vi "DCS_Dual_Inst.vi"(3 "error in":errorcluster) -> (10 "error out":errorcluster)   [LabVIEW 2013]
uses:
  <vilib>/Utility/miscctls.llb/LVPointTypeDef.ctl
  Controls/Role ID.ctl
panel:
  out "Changed front panel":bool
  in  "stop":bool
  in  "Tab Control":enum32{"Engineering Graphs", "Maintenance"}(tab)
  out "DCS 2 Second Plane":ext[][](graph)
  out "DCS 2 First Plane":ext[][](graph)
  out "DCS 1 Second Plane":ext[][](graph)
  out "DCS 1 First Plane":ext[][](graph)
  out "DCS 1 Signals":dbl[][](graph)
  out "DCS 2 Signals":dbl[][](graph)
  in  "Save Waveforms":bool
  in  "Minimum Particle Velocity (km/s)":dbl=3.0
  in  "Use Partical Veloctiy":bool=TRUE
  out "Aquisition Rate Value 2":i64
  out "Aquisition Rate Value 1":i64
  out "DAQ 1 Sample Size Window":u32
  in  "DAQ 1 Trim Time":dbl=0.0001
  in  "DAQ 2 Trim Time":dbl=0.0001
  out "DAQ 2 Sample Size Window":i32
  in  "Posttrigger size 2":i32=5000
  in  "Acquisition Rate 2":u16(ring) items=["40 MHz", "20 MHz", "10 MHz", "5 MHz", "2.5 MHz", "1 MHz", "100 kHz", "10 kHz"]
  in  "Pretrigger size 2":i32=1
  in  "Rising or falling? 2":bool
  in  "Jorger 2 TR slot":i32=6
  out "Sampling Frequency":u16(ring) items=["40 MHz", "20 MHz", "10 MHz", "5 MHz", "2.5 MHz", "1 MHz", "100 kHz", "10 kHz"]
  out "Length of Sample":dbl caption="s" format="%^#_3g"
  out "Memory Address Pointer":ext
  out "Post trigger Size":ext
  out "Pretrigger Size":ext
  out "Trigger Generation register":i32=23 format="%.0b"
  out "status register":i8=4 format="%08b"
  out "control register":i16=23 format="%015b"
  in  "Posttrigger size":i32=1
  in  "Acquisition Rate":u16(ring) items=["40 MHz", "20 MHz", "10 MHz", "5 MHz", "2.5 MHz", "1 MHz", "100 kHz", "10 kHz"]
  in  "Pretrigger size":i32=15000
  in  "Rising or falling?":bool
  out "Running Errors":errorcluster
  in  "Jorger 1 TR slot":i32=3
  in  "Joerger 1 Channels":i32[](array[numeric])=[0, 1, 2, 3, 4, 5, 6, 9]
  in  "Joerger 2 Channels":i32[](array[numeric])=[0, 1, 2, 3, 4, 6, 7, 8]
  out "control register 2":i16=23 format="%015b"
  out "status register 2":i8=4 format="%08b"
  out "Memory Address Pointer 2":ext
  out "Post trigger Size 2":ext
  out "Pretrigger Size 2":ext
  out "Sampling Frequency 2":u16(ring) items=["40 MHz", "20 MHz", "10 MHz", "5 MHz", "2.5 MHz", "1 MHz", "100 kHz", "10 kHz"]
  out "DCS_1_Pre_Trigger":dbl
  out "DCS_2_Post_Trigger":dbl
  # "Ensure Joeger Card Channels are functional.\nDefault values should reflect this."
  # "Rising or falling? not functional. Ignore"
  # "DAQ 2 Parameter Controls"
  # "Falling"
  # "Rising"
  # "DAQ Parameter Indicators"
  # "DAQ 1 Parameter Controls"
  # "Falling"
  # "Rising"
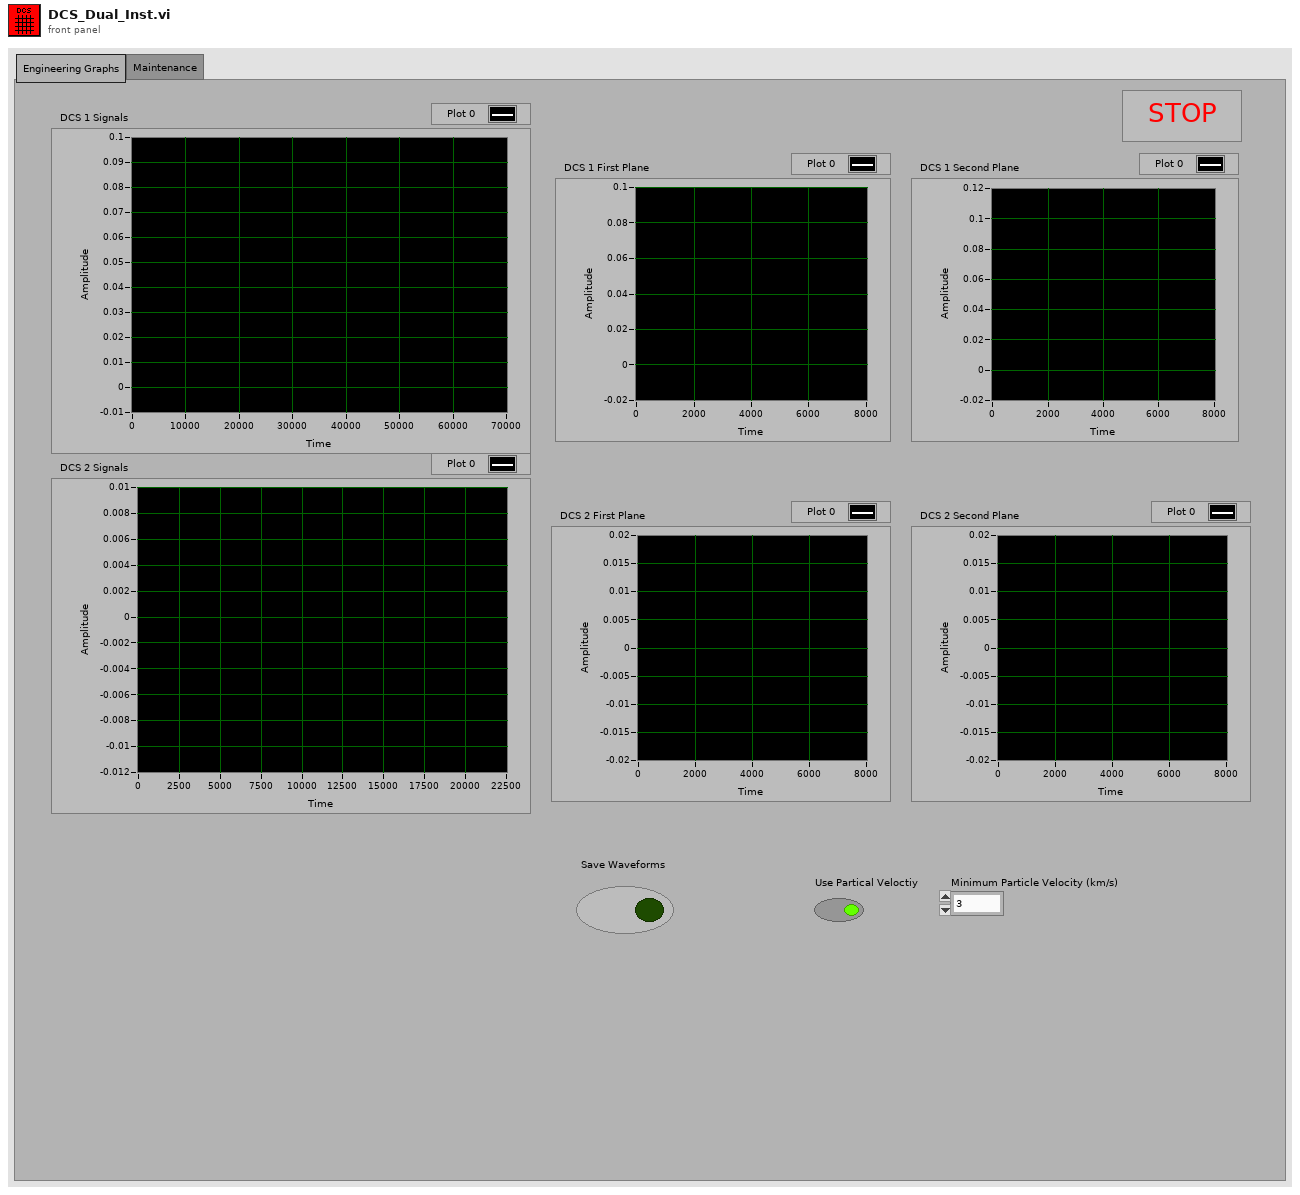
[diagram p1: front panel]
types:
  T1 = typedef "LVPointTypeDef.ctl" = cluster{"Horizontal":i16, "Vertical":i16}
  T2 = typedef "Role ID.ctl" = enum16{"First_Detector", "Second_Detector", "Third_Detector", "LeCroy_CH1", "LeCroy_CH2", "LeCroy_CH3", "LeCroy_CH4", "PSU", "DCS 1", "DCS 2"}
  T3 = enum32{"DCS", "Spot Size Tracking", "Engineering Graphs", "Maintenance"}
  T4 = cluster{"Data":dbl[][], "Integer Timestamp":u64, "Signal Length":u32, "DCS ID":u64, "Role ID":T2, "Aquisition Rate":dbl}
  T5 = cluster{"Data":dbl[][], "Integer Timestamp":u64, "Signal Length":u32, "DCS ID":u64, "Role ID":T2, "Aquisition Rate":dbl}[]
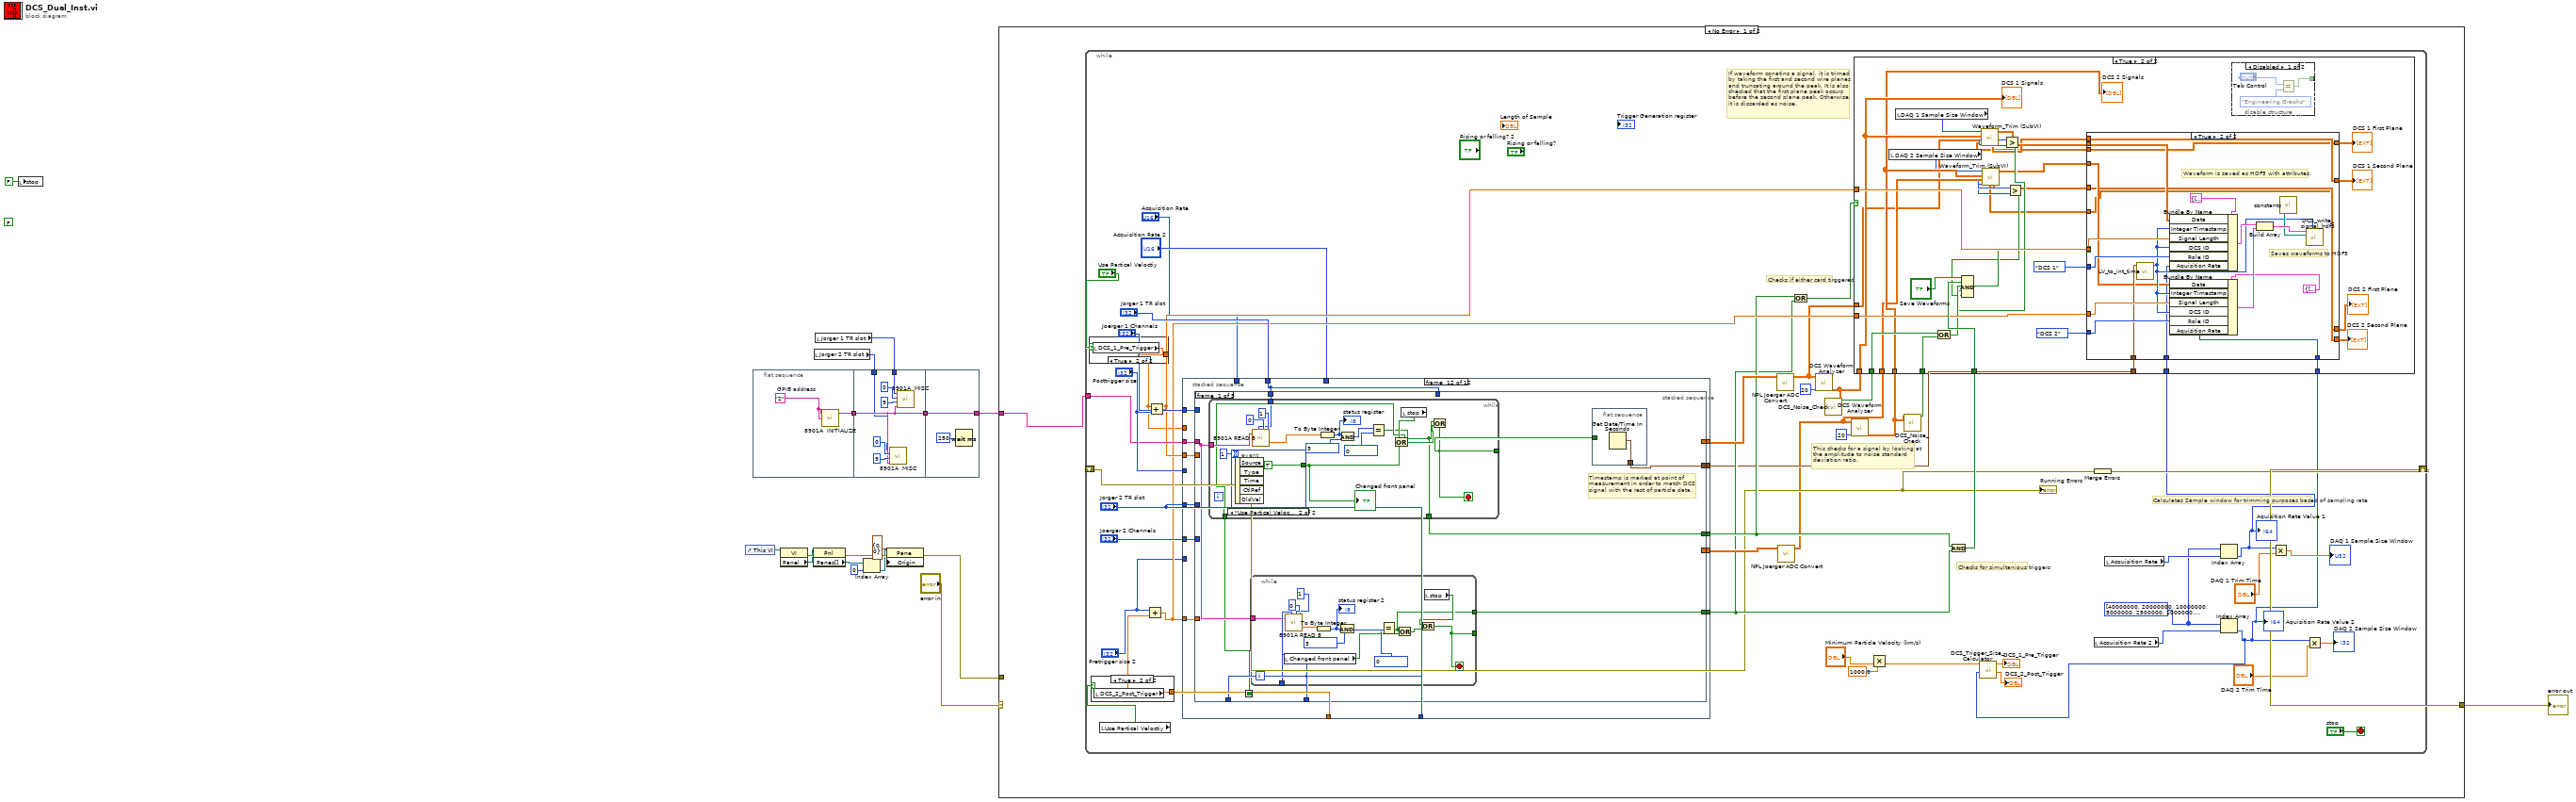
[diagram p0: block diagram]
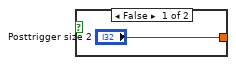
[diagram p2: hidden frame]
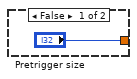
[diagram p3: hidden frame]
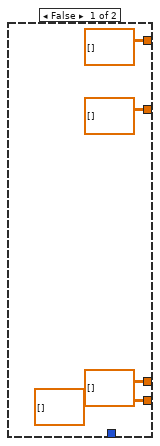
[diagram p6: hidden frame]
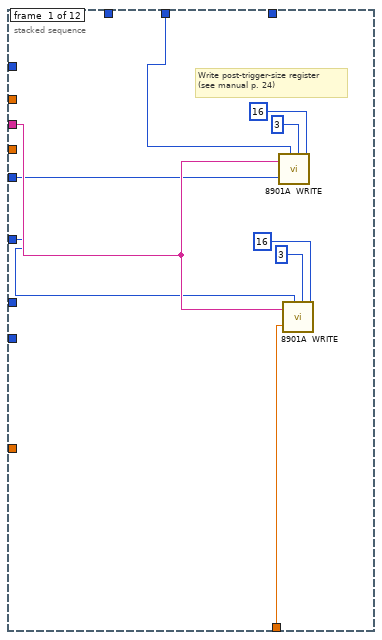
[diagram p7: hidden frame]
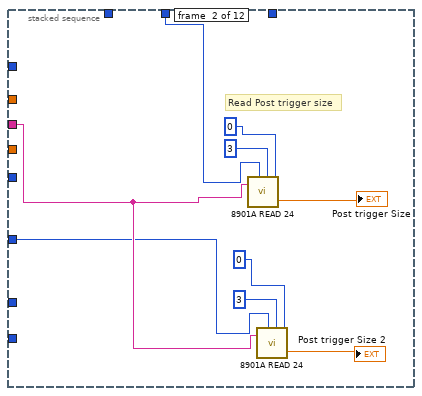
[diagram p8: hidden frame]
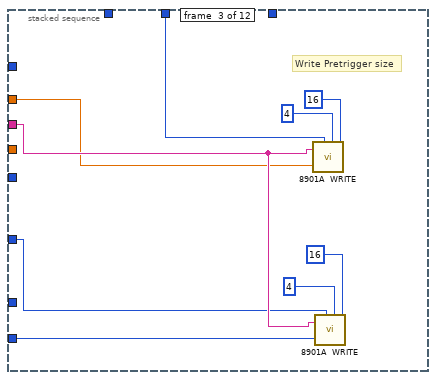
[diagram p9: hidden frame]
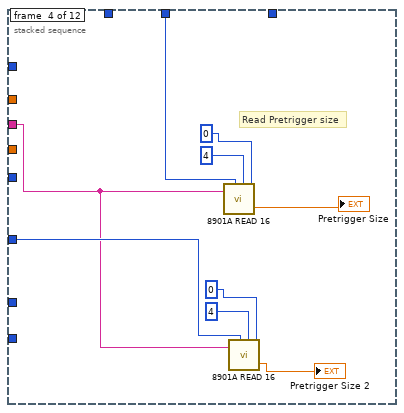
[diagram p10: hidden frame]
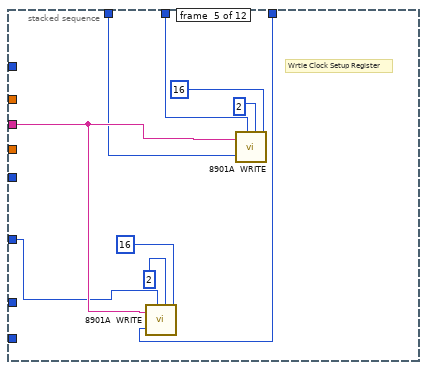
[diagram p11: hidden frame]
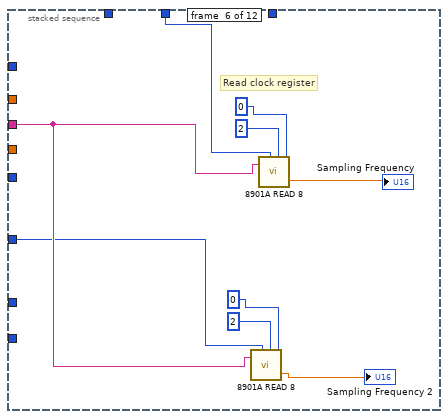
[diagram p12: hidden frame]
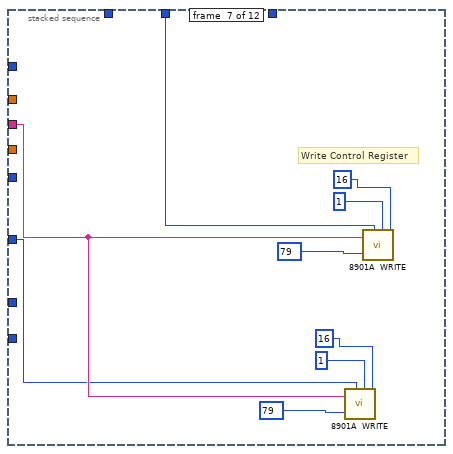
[diagram p13: hidden frame]
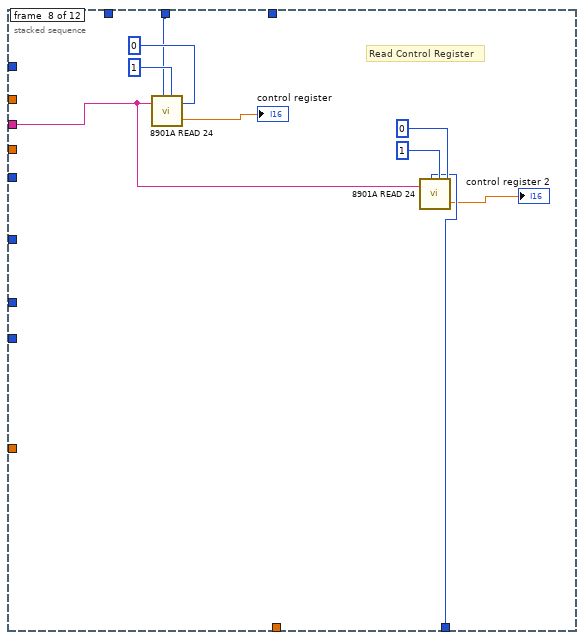
[diagram p14: hidden frame]
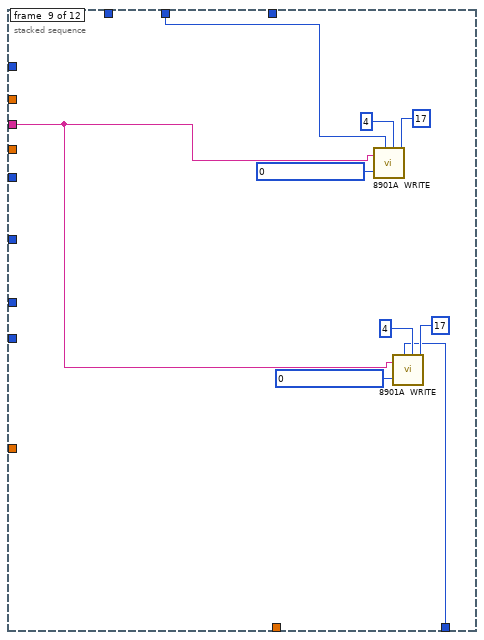
[diagram p15: hidden frame]
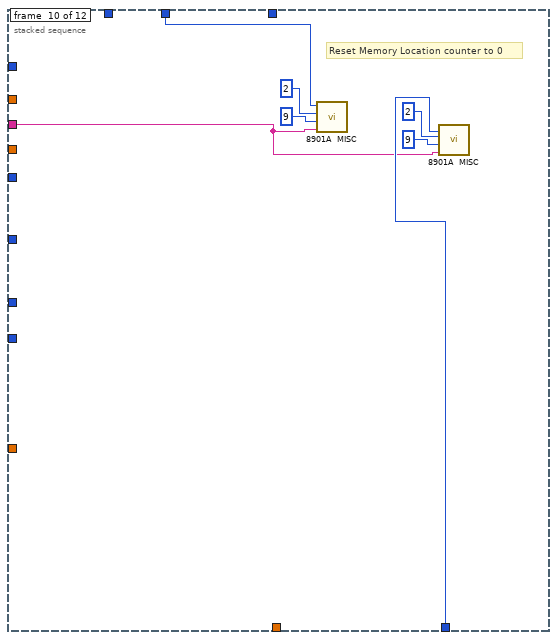
[diagram p16: hidden frame]
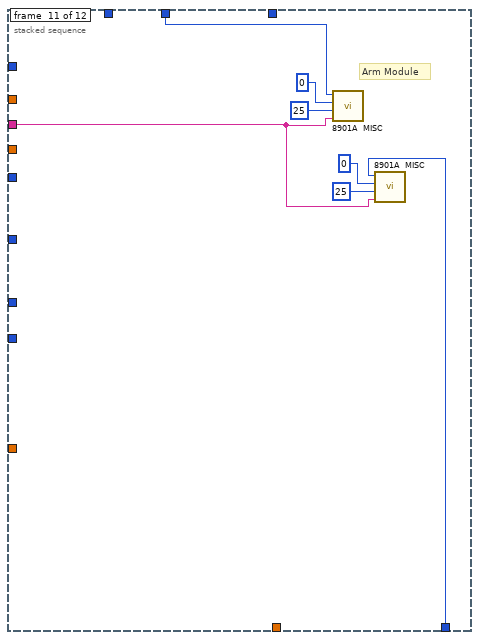
[diagram p17: hidden frame]
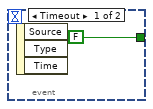
[diagram p18: hidden frame]
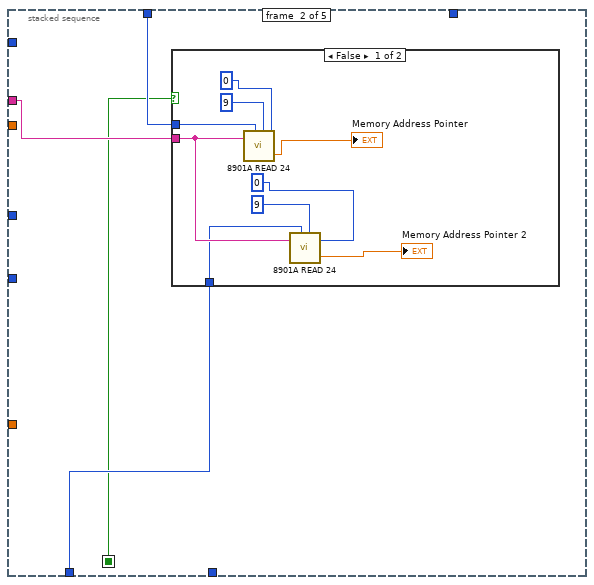
[diagram p19: hidden frame]
diagram:
  (unwired) FALSE ("Auto Threshold")
  n1 = local write "stop"(FALSE ("stop")) -> ()
  n2 = control-ref of="This VI"() -> (w14:refnum<vi>)
  n3 = flat-sequence {
    tunnel: [w18] -> w4
    tunnel: w4 -> [w21]
    tunnel: w3 -> [w20]
    tunnel: w2 -> [w19]
    tunnel: [w21] -> w1
    tunnel: [w27] -> w5
    tunnel: w1 -> [w27]
    frame #0 {
      w18 = "2"  # GPIB address
      n4 = call <instrlib>:"8901A  INITIALIZE.vi"("GPIB address"=w18) -> ()
    }
    frame #1 {
      n5 = call <instrlib>:"8901A  MISC.vi"("GPIB address"=w21, "f"=9, "a"=0, "n"=w19) -> ()
      n6 = call <instrlib>:"8901A  MISC.vi"("GPIB address"=w21, "f"=9, "a"=0, "n"=w20) -> ()
    }
    frame #2 {
      n7 = Wait (ms)(milliseconds to wait=250) -> ()  [unwired: 1 out]
    }
  }
  n8 = property class="VI"(reference=w14) -> (error out=w13:errorcluster, "Panel"=w12:refnum<vi>)  [unwired: 1 in, 1 out]
  n9 = property class="Pnl"(reference=w12, error in=w13) -> (error out=w11:errorcluster, "Panes[]"=w10:refnum<vi>[])  [unwired: 1 out]
  n10 = local read "Jorger 2 TR slot"() -> (w2:i32)
  n11 = local read "Jorger 1 TR slot"() -> (w3:i32)
  n12 = Index Array(array=w10, index=0) -> (element=w8:refnum<vi>)
  n13 = property class="Pane"(reference=w8, error in=w11, "Origin"=T1 {"Horizontal"=0, "Vertical"=0}) -> (error out=w6:errorcluster)  [unwired: 1 out]
  n14 = case shown="No Error" "error in" {
    selector: "error in" -> [_ w380]
    tunnel: [w29 w380] -> w16
    tunnel: w6 -> [_ _]
    tunnel: w5 -> [w28 _]
    frame No Error {
      n15 = while {
        shift-right: [w47] -> w29
        shift-left: _ -> [w48]
        tunnel: w28 -> [w68]
        stop <- "stop" stop-if-true
        w51 = i32[] [40000000, 20000000, 10000000, 5000000, 2500000, 1000000, 100000, 10000]
        # "This checks for a signal by looking at the amplitude to noise standard deviation ratio."
        # "If waveform conatins a signal, it is trimed\nby taking the first and second wire planes\nand truncating around the peak. It is also \nchecked that the first plane peak occurs\nbefore the second plane peak. Otherwise, \nit is discarded as noise."
        # "Calculates Sample window for trimming purposes based of sampling rate"
        # "Checks if either card tirggered"
        # "Checks for simultanious triggers"
        n16 = case shown="True" "Use Partical Veloctiy" {
          tunnel: ["Pretrigger size" w80] -> w58
          frame False {
          }
          frame True {
            n17 = local read "DCS_1_Pre_Trigger"() -> (w80:dbl)
          }
        }
        n18 = local read "Use Partical Veloctiy"() -> (w36:bool)
        n19 = case shown="True" w36 {
          tunnel: ["Posttrigger size 2" w78] -> w70
          frame False {
          }
          frame True {
            n20 = local read "DCS_2_Post_Trigger"() -> (w78:dbl)
          }
        }
        n21 = Add(x="Pretrigger size 2", y=w70) -> (x+y=w65:dbl)
        n22 = Add(x=w58, y="Posttrigger size") -> (x+y=w66:dbl)
        n23 = stacked-sequence {
          tunnel: w68 -> [w147 w158 w165 w170 w183 w194 w198 w209 w217 w229 w233 w247]
          tunnel: w66 -> [_ _ _ _ _ _ _ _ _ _ _ w250]
          tunnel: "Joerger 1 Channels" -> [_ _ _ _ _ _ _ _ _ _ _ w249]
          tunnel: [_ _ _ _ _ _ _ _ _ _ _ w248] -> w74
          tunnel: "Jorger 2 TR slot" -> [_ _ _ _ _ _ _ w208 w215 w230 w232 w246]
          tunnel: "Jorger 1 TR slot" -> [w146 w154 w164 w174 w182 w192 w202 w206 w216 w228 w231 w239]
          tunnel: "Jorger 2 TR slot" -> [w145 w155 w163 w173 w181 w191 w197 _ _ _ _ w244]
          tunnel: "Posttrigger size" -> [w144 _ _ _ _ _ _ _ _ _ _ _]
          tunnel: w70 -> [w143 _ _ _ _ _ _ _ _ _ _ _]
          tunnel: "Acquisition Rate" -> [_ _ _ _ w180 _ _ _ _ _ _ _]
          tunnel: "Acquisition Rate 2" -> [_ _ _ _ w179 _ _ _ _ _ _ _]
          tunnel: w65 -> [_ _ _ _ _ _ _ _ _ _ _ w245]
          tunnel: "Joerger 2 Channels" -> [_ _ _ _ _ _ _ _ _ _ _ w243]
          tunnel: [_ _ _ _ _ _ _ _ _ _ _ w242] -> w67
          tunnel: [_ _ _ _ _ _ _ _ _ _ _ w241] -> w63
          tunnel: [_ _ _ _ _ _ _ _ _ _ _ w240] -> w62
          tunnel: "Pretrigger size 2" -> [_ _ w162 _ _ _ _ _ _ _ _ _]
          tunnel: w58 -> [_ _ w161 _ _ _ _ _ _ _ _ _]
          tunnel: [_ _ _ _ _ _ _ _ _ _ _ w238] -> w56
          frame #0 {
            # "Write post-trigger-size register\n(see manual p. 24)"
            n24 = call <instrlib>:"8901A  WRITE.vi"("data"=w144, "GPIB address"=w147, "n"=w146, "a"=3, "f"=16) -> ()  [unwired: 1 in]
            n25 = call <instrlib>:"8901A  WRITE.vi"("data"=w143, "GPIB address"=w147, "n"=w145, "a"=3, "f"=16) -> ()  [unwired: 1 in]
          }
          frame #1 {
            # "Read Post trigger size"
            n26 = call <instrlib>:"8901A READ 24.vi"("GPIB address"=w158, "n"=w154, "a"=3, "f"=0) -> ("output"=→"Post trigger Size":ext)  [unwired: 3 in]
            n27 = call <instrlib>:"8901A READ 24.vi"("GPIB address"=w158, "n"=w155, "a"=3, "f"=0) -> ("output"=→"Post trigger Size 2":ext)  [unwired: 3 in]
          }
          frame #2 {
            # "Write Pretrigger size"
            n28 = call <instrlib>:"8901A  WRITE.vi"("data"=w161, "GPIB address"=w165, "n"=w164, "a"=4, "f"=16) -> ()  [unwired: 1 in]
            n29 = call <instrlib>:"8901A  WRITE.vi"("data"=w162, "GPIB address"=w165, "n"=w163, "a"=4, "f"=16) -> ()  [unwired: 1 in]
          }
          frame #3 {
            # "Read Pretrigger size"
            n30 = call <instrlib>:"8901A READ 16.vi"("GPIB address"=w170, "n"=w174, "a"=u8 4, "f"=u8 0) -> ("output"=→"Pretrigger Size":ext)  [unwired: 3 in]
            n31 = call <instrlib>:"8901A READ 16.vi"("GPIB address"=w170, "n"=w173, "a"=u8 4, "f"=u8 0) -> ("output"=→"Pretrigger Size 2":ext)  [unwired: 3 in]
          }
          frame #4 {
            # "Wrtie Clock Setup Register"
            n32 = call <instrlib>:"8901A  WRITE.vi"("data"=w179, "GPIB address"=w183, "n"=w181, "a"=2, "f"=16) -> ()  [unwired: 1 in]
            n33 = call <instrlib>:"8901A  WRITE.vi"("data"=w180, "GPIB address"=w183, "n"=w182, "a"=2, "f"=16) -> ()  [unwired: 1 in]
          }
          frame #5 {
            # "Read clock register"
            n34 = call <instrlib>:"8901A READ 8.vi"("GPIB address"=w194, "n"=w191, "a"=2, "f"=0) -> ("output"=→"Sampling Frequency 2":ext)  [unwired: 3 in]
            n35 = call <instrlib>:"8901A READ 8.vi"("GPIB address"=w194, "n"=w192, "a"=2, "f"=0) -> ("output"=→"Sampling Frequency":ext)  [unwired: 3 in]
          }
          frame #6 {
            # "Write Control Register"
            n36 = call <instrlib>:"8901A  WRITE.vi"("data"=79, "GPIB address"=w198, "n"=w197, "a"=1, "f"=16) -> ()  [unwired: 1 in]
            n37 = call <instrlib>:"8901A  WRITE.vi"("data"=79, "GPIB address"=w198, "n"=w202, "a"=1, "f"=16) -> ()  [unwired: 1 in]
          }
          frame #7 {
            # "Read Control Register"
            n38 = call <instrlib>:"8901A READ 24.vi"("GPIB address"=w209, "n"=w206, "a"=1, "f"=0) -> ("output"=→"control register":ext)  [unwired: 3 in]
            n39 = call <instrlib>:"8901A READ 24.vi"("GPIB address"=w209, "n"=w208, "a"=1, "f"=0) -> ("output"=→"control register 2":ext)  [unwired: 3 in]
          }
          frame #8 {
            n40 = call <instrlib>:"8901A  WRITE.vi"("data"=0, "GPIB address"=w217, "n"=w216, "a"=u8 4, "f"=u8 17) -> ()  [unwired: 1 in]
            n41 = call <instrlib>:"8901A  WRITE.vi"("data"=0, "GPIB address"=w217, "n"=w215, "a"=u8 4, "f"=u8 17) -> ()  [unwired: 1 in]
          }
          frame #9 {
            # "Reset Memory Location counter to 0"
            n42 = call <instrlib>:"8901A  MISC.vi"("GPIB address"=w229, "f"=u8 9, "a"=u8 2, "n"=w228) -> ()
            n43 = call <instrlib>:"8901A  MISC.vi"("GPIB address"=w229, "f"=u8 9, "a"=u8 2, "n"=w230) -> ()
          }
          frame #10 {
            # "Arm Module"
            n44 = call <instrlib>:"8901A  MISC.vi"("GPIB address"=w233, "f"=25, "a"=0, "n"=w231) -> ()
            n45 = call <instrlib>:"8901A  MISC.vi"("GPIB address"=w233, "f"=25, "a"=0, "n"=w232) -> ()
          }
          frame #11 {
            n46 = stacked-sequence {
              seq-local: [w256 _ _ _ _] -> [_ w291 w313 _ _]
              tunnel: w250 -> [_ _ w312 _ _]
              tunnel: w249 -> [_ _ w311 _ _]
              tunnel: [_ _ w309 _ _] -> w248
              tunnel: w246 -> [w258 _ _ w365 _]
              tunnel: w247 -> [w257 w294 w310 w366 w375]
              tunnel: w246 -> [_ w293 _ _ _]
              tunnel: w245 -> [_ _ w308 _ _]
              tunnel: w239 -> [_ _ w307 _ w374]
              tunnel: w244 -> [_ _ w305 _ w373]
              tunnel: w243 -> [_ _ w306 _ _]
              tunnel: [_ _ w304 _ _] -> w242
              tunnel: [w255 _ _ _ _] -> w241
              tunnel: [w254 _ _ _ _] -> w240
              tunnel: w239 -> [w253 w292 _ w369 _]
              tunnel: [w251 _ _ _ _] -> w238
              frame #0 {
                # "Timestamp is marked at point of \nmeasurement in order to match DCS\nsignal with the rest of particle data."
                n47 = while {
                  tunnel: w257 -> [w281]
                  tunnel: [w279] -> w252
                  tunnel: [w275] -> w256
                  tunnel: [w274] -> w255
                  tunnel: w253 -> [w273]
                  stop <- w279 stop-if-true
                  n48 = event shown="[1] \"Use Partical Veloctiy\", \"Acquisition Rate\", \"Posttrigger size\", \"control register\", \"Minimum Particle Velocity (km/s)\": Value Change" {
                    selector: _ -> [_ _]
                    dyn-events: _ -> [_ _]
                    timeout: 1 -> [_ _]
                    tunnel: [FALSE TRUE] -> w277
                    event Timeout {
                      n49 = event-data() -> ()  [unwired: 1 in, 3 out]
                    }
                    event "Use Partical Veloctiy", "Acquisition Rate", "Posttrigger size", "control register", "Minimum Particle Velocity (km/s)": Value Change {
                      n50 = event-data() -> ()  [unwired: 1 in, 5 out]
                    }
                  }
                  "Changed front panel" <- w277
                  n51 = call <instrlib>:"8901A READ 8.vi"("GPIB address"=w281, "n"=w273, "a"=0, "f"=1) -> ("output"=w284:ext)  [unwired: 3 in]
                  n52 = To Byte Integer(number=w284) -> (8bit integer=w280:i8)
                  "status register" <- w280
                  n53 = And(x=w280, y=i8 3) -> (x .and. y?=w285:i8)
                  n54 = Equal?(x=w285, y=i8 0) -> (x = y?=w274:bool)
                  n55 = local read "stop"() -> (w276:bool)
                  n56 = Or(x=w276, y=w277) -> (x .or. y?=w275:bool)
                  n57 = Or(x=w274, y=w275) -> (x .or. y?=w279:bool)
                }
                n58 = while {
                  tunnel: w258 -> [w270]
                  tunnel: w257 -> [w269]
                  tunnel: [w262] -> _
                  tunnel: [w259] -> w254
                  stop <- w262 stop-if-true
                  n59 = local read "Changed front panel"() -> (w260:bool)
                  n60 = call <instrlib>:"8901A READ 8.vi"("GPIB address"=w269, "n"=w270, "a"=0, "f"=1) -> ("output"=w268:ext)  [unwired: 3 in]
                  n61 = To Byte Integer(number=w268) -> (8bit integer=w264:i8)
                  "status register 2" <- w264
                  n62 = And(x=w264, y=i8 3) -> (x .and. y?=w266:i8)
                  n63 = Equal?(x=w266, y=i8 0) -> (x = y?=w259:bool)
                  n64 = Or(x=w259, y=w260) -> (x .or. y?=w261:bool)
                  n65 = local read "stop"() -> (w263:bool)
                  n66 = Or(x=w263, y=w261) -> (x .or. y?=w262:bool)
                }
                n67 = flat-sequence {
                  tunnel: w252 -> [_]
                  tunnel: [w290] -> w251
                  frame #0 {
                    n68 = Get Date/Time In Seconds() -> (seconds since 1Jan1904=w290:timestamp)
                  }
                }
              }
              frame #1 {
                n69 = case shown="False" w291 {
                  tunnel: w294 -> [w298 _]
                  tunnel: w293 -> [w297 _]
                  tunnel: w292 -> [w295 _]
                  frame False {
                    n70 = call <instrlib>:"8901A READ 24.vi"("GPIB address"=w298, "n"=w295, "a"=u8 9, "f"=u8 0) -> ("output"=→"Memory Address Pointer":ext)  [unwired: 3 in]
                    n71 = call <instrlib>:"8901A READ 24.vi"("GPIB address"=w298, "n"=w297, "a"=u8 9, "f"=u8 0) -> ("output"=→"Memory Address Pointer 2":ext)  [unwired: 3 in]
                  }
                  frame True {
                  }
                }
              }
              frame #2 {
                n72 = case shown="False" w313 {
                  tunnel: w312 -> [w323 _]
                  tunnel: w311 -> [w324 _]
                  tunnel: w310 -> [w322 _]
                  tunnel: [w320 ext[][] [[nan]] ("output")] -> w309
                  tunnel: w308 -> [w319 _]
                  tunnel: w307 -> [w317 _]
                  tunnel: w305 -> [w316 _]
                  tunnel: w306 -> [w315 _]
                  tunnel: [w314 ext[][] [[nan]] ("output")] -> w304
                  frame False {
                    n73 = local read "Memory Address Pointer 2"() -> (w318:ext)
                    n74 = local read "Memory Address Pointer"() -> (w321:ext)
                    n75 = for {
                      N: 8 -> [_]
                      tunnel: w324 -> [w337] mode=indexing
                      tunnel: w323 -> [w328]
                      tunnel: w322 -> [w339]
                      tunnel: w321 -> [w341]
                      tunnel: [w336] -> w320 mode=indexing
                      tunnel: w319 -> [w334]
                      tunnel: w318 -> [w335]
                      tunnel: w317 -> [w332]
                      tunnel: w316 -> [w331]
                      tunnel: w315 -> [w327] mode=indexing
                      tunnel: [w326] -> w314 mode=indexing
                      n76 = Subtract(x=w341, y=w328) -> (x-y=w340:ext)
                      n77 = Subtract(x=w335, y=w334) -> (x-y=w333:ext)
                      n78 = flat-sequence {
                        tunnel: w340 -> [w348]
                        tunnel: w339 -> [w346]
                        tunnel: [w346] -> w338
                        tunnel: w333 -> [w347]
                        tunnel: w332 -> [w342]
                        tunnel: w331 -> [w343]
                        tunnel: [w342] -> w330
                        tunnel: [w343] -> w329
                        tunnel: w338 -> [w354]
                        tunnel: w337 -> [w356]
                        tunnel: w328 -> [w360]
                        tunnel: [w359] -> w336
                        tunnel: w334 -> [w357]
                        tunnel: w330 -> [w351]
                        tunnel: w329 -> [w352]
                        tunnel: w327 -> [w355]
                        tunnel: [w353] -> w326
                        frame #0 {
                          n79 = call <instrlib>:"8901A  WRITE.vi"("data"=w348, "GPIB address"=w346, "n"=w342, "a"=1, "f"=17) -> ()  [unwired: 1 in]
                          n80 = call <instrlib>:"8901A  WRITE.vi"("data"=w347, "GPIB address"=w346, "n"=w343, "a"=1, "f"=17) -> ()  [unwired: 1 in]
                        }
                        frame #1 {
                          n81 = call <instrlib>:"8901A BLOCK READ 24.vi"("f"=2, "a"=w356, "n"=w351, "GPIB address"=w354, "# points to read"=w360) -> ("output"=w359:ext[])  [unwired: 4 in]
                          n82 = call <instrlib>:"8901A BLOCK READ 24.vi"("f"=2, "a"=w355, "n"=w352, "GPIB address"=w354, "# points to read"=w357) -> ("output"=w353:ext[])  [unwired: 4 in]
                        }
                      }
                    }
                  }
                  frame True {
                  }
                }
              }
              frame #3 {
                # "Read in control register"
                n83 = call <instrlib>:"8901A READ 24.vi"("GPIB address"=w366, "n"=w369, "a"=1, "f"=0) -> ("output"=w370:ext)  [unwired: 3 in]
                n84 = call <instrlib>:"8901A READ 24.vi"("GPIB address"=w366, "n"=w365, "a"=1, "f"=0) -> ("output"=w364:ext)  [unwired: 3 in]
                n85 = local write "control register"(w370) -> ()
                n86 = local write "control register 2"(w364) -> ()
              }
              frame #4 {
                # "Abort Readout"
                n87 = call <instrlib>:"8901A  MISC.vi"("GPIB address"=w375, "f"=25, "a"=2, "n"=w373) -> ()
                n88 = call <instrlib>:"8901A  MISC.vi"("GPIB address"=w375, "f"=25, "a"=2, "n"=w374) -> ()
              }
            }
          }
        }
        n89 = call "NPL Joerger ADC Convert.vi"("Input"=w74) -> ("Output"=w33:ext[][])  [unwired: 10 in]
        n90 = call "NPL Joerger ADC Convert.vi"("Input"=w67) -> ("Output"=w32:ext[][])  [unwired: 10 in]
        n91 = Or(x=w63, y=w62) -> (x .or. y?=w61:bool)
        n92 = call "DCS Waveform Analyzer.vi"("Rank"=20, "8 DCS Waveforms"=w33) -> ("Filtered Signals"=w42:dbl[][])  [unwired: 8 in, 1 out]
        n93 = call "DCS_Noise_Check.vi"("8 DCS Waveforms"=w42) -> ("Boolean"=w41:bool)  [unwired: 10 in]
        n94 = call "DCS Waveform Analyzer.vi"("Rank"=20, "8 DCS Waveforms"=w32) -> ("Filtered Signals"=w44:dbl[][])  [unwired: 8 in, 1 out]
        n95 = Multiply(x=1000.0, y="Minimum Particle Velocity (km/s)") -> (x*y=w35:dbl)
        n96 = call "DCS_Noise_Check.vi"("8 DCS Waveforms"=w44) -> ("Boolean"=w43:bool)  [unwired: 10 in]
        n97 = And(x=w63, y=w62) -> (x .and. y?=w64:bool)
        n98 = Merge Errors(w48) -> (w47:errorcluster)
        n99 = local read "Acquisition Rate 2"() -> (w53:u16)
        n100 = local read "Acquisition Rate"() -> (w52:u16)
        n101 = Index Array(array=w51, index=w52) -> (element=w31:i32)
        "Aquisition Rate Value 1" <- w31
        n102 = Index Array(array=w51, index=w53) -> (element=w30:i32)
        "Aquisition Rate Value 2" <- w30
        n103 = case shown="True" w61 {
          tunnel: w42 -> [_ w100]
          tunnel: w66 -> [_ w114]
          tunnel: w44 -> [_ w95]
          tunnel: w64 -> [_ w111]
          tunnel: w65 -> [_ w110]
          tunnel: w56 -> [_ w109]
          tunnel: w43 -> [_ w108]
          tunnel: w41 -> [_ w107]
          tunnel: w33 -> [_ w86]
          tunnel: w32 -> [_ w94]
          tunnel: w31 -> [_ w82]
          tunnel: w30 -> [_ w81]
          frame False {
          }
          frame True {
            n104 = local read "DAQ 2 Sample Size Window"() -> (w93:i32)
            n105 = local read "DAQ 1 Sample Size Window"() -> (w99:u32)
            n106 = Or(x=w107, y=w108) -> (x .or. y?=w105:bool)
            n107 = call "Waveform_Trim (SubVI).vi"("Raw Waveform"=w86, "Filtered Waveform"=w100, "DAQ Sample Window"=w99) -> ("Second Plane Max Value Index"=w98:i32, "First Plane Max Value Index"=w97:i32, "Trimmed Waveform"=w89:ext[][], "Second Plane"=w88:ext[][], "First Plane"=w87:ext[][])  [unwired: 4 in]
            n108 = call "Waveform_Trim (SubVI).vi"("Raw Waveform"=w94, "Filtered Waveform"=w95, "DAQ Sample Window"=w93) -> ("Second Plane Max Value Index"=w92:i32, "First Plane Max Value Index"=w91:i32, "Trimmed Waveform"=w85:ext[][], "Second Plane"=w84:ext[][], "First Plane"=w83:ext[][])  [unwired: 4 in]
            n109 = Greater?(x=w98, y=w97) -> (0:w96:bool)
            n110 = Greater?(x=w92, y=w91) -> (0:w90:bool)
            n111 = Compound Arithmetic op=AND("Save Waveforms", w111, w105, w96, w90) -> (w106:bool)
            n112 = case shown="True" w106 {
              tunnel: Role_ID."DCS 1" ("Role ID") -> [_ w140]
              tunnel: w114 -> [_ w139]
              tunnel: w110 -> [_ w137]
              tunnel: Role_ID."DCS 2" ("Role ID") -> [_ w136]
              tunnel: w109 -> [_ w135]
              tunnel: [ext[][] [] ("First Plane") w130] -> w104
              tunnel: [ext[][] [] ("Second Plane") w131] -> w103
              tunnel: [ext[][] [] ("Second Plane") w128] -> w102
              tunnel: [ext[][] [] ("First Plane") w127] -> w101
              tunnel: w89 -> [_ w132]
              tunnel: w88 -> [_ w131]
              tunnel: w87 -> [_ w130]
              tunnel: w85 -> [_ w129]
              tunnel: w84 -> [_ w128]
              tunnel: w83 -> [_ w127]
              tunnel: w82 -> [_ w124]
              tunnel: w81 -> [_ w123]
              frame False {
              }
              frame True {
                # "Waveform is saved as HDF5 with attributes."
                # "Saves waveforms to HDF5"
                n113 = call "LV_to_int_time.vi"("Time Stamp"=w135) -> ("Integer Time"=w133:i64)  [unwired: 8 in, 1 out]
                n114 = Bundle By Name(cluster=T4 {"Data"=[], "Integer Timestamp"=0, "Signal Length"=0, "DCS ID"=0, "Role ID"=enum."First_Detector", "Aquisition Rate"=0.0} ("Cluster"), "Data"=w132, "Integer Timestamp"=w133, "Signal Length"=w139, "DCS ID"=w133, "Role ID"=w140, "Aquisition Rate"=w124) -> (w142:T4)
                n115 = Bundle By Name(cluster=T4 {"Data"=[], "Integer Timestamp"=0, "Signal Length"=0, "DCS ID"=0, "Role ID"=enum."First_Detector", "Aquisition Rate"=0.0} ("Cluster"), "Data"=w129, "Integer Timestamp"=w133, "Signal Length"=w137, "DCS ID"=w133, "Role ID"=w136, "Aquisition Rate"=w123) -> (w138:T4)
                n116 = Build Array(w142, w138) -> (w141:T5)
                n117 = call "constants.vi"() -> ("DCS Temp filepath"=w134:path)  [unwired: 3 out]
                n118 = call "DCS_write_signal_hdf5.vi"("Index"=w133, "Save Path"=w134, "Signal array"=w141) -> ()  [unwired: 8 in, 1 out]
              }
            }
            "DCS 1 First Plane" <- w104
            "DCS 1 Second Plane" <- w103
            "DCS 2 Second Plane" <- w102
            "DCS 2 First Plane" <- w101
            n119 = disable-structure shown="Disabled" {
              disable-tunnel: [w116 _] -> _
              frame Disabled {
                n120 = Equal?(x="Tab Control", y=T3."Engineering Graphs") -> (x = y?=w116:bool)
              }
              frame Enabled {
              }
            }
            "DCS 1 Signals" <- w100
            "DCS 2 Signals" <- w95
          }
        }
        n121 = call "DCS_Trigger_Size_Calculator.vi"("Sample_Rate (Hz)"=w30, "Partical_Velocity (m/s)"=w35) -> ("DCS_2_Post_Trigger"=→"DCS_2_Post_Trigger":dbl, "DCS_1_Pre_Trigger"=→"DCS_1_Pre_Trigger":dbl)  [unwired: 8 in]
        n122 = Multiply(x=w31, y="DAQ 1 Trim Time") -> (x*y=→"DAQ 1 Sample Size Window":dbl)
        n123 = Multiply(x=w30, y="DAQ 2 Trim Time") -> (x*y=→"DAQ 2 Sample Size Window":dbl)
        "Running Errors" <- w48
      }
    }
    frame Error {
    }
  }
  "error out" <- w16
